vi "בדיקת מפל מתח בין הדקי הממסר תחת עומס Mod.vi"(6 "זרם הדרוש":sgl=20.0, 8 "error":errorcluster, 9 "מפל מתח מקסימלי":dbl=0.205 format="%#_13g", 10 "שם הממסר":string="0410-24534 15A ממסר", 11 "Path for Log":path) -> (0 "error IO":errorcluster, 1 "In Range?":bool, 2 "מפל מתח בין דקי הממסר תחת עומס":dbl, 3 "תוצאה זמנית":dbl)   [LabVIEW 2014]
uses:
  M9700 Driver/86/vi.lib/M9700 Modbus.llb/CTL CMD Register.ctl
  M9700 Driver/85/vi.lib/M9700 Modbus.llb/CTL Register Address.ctl
  <vilib>/Instr/_visa.llb/VISA Configure Serial Port (Instr).vi
  <vilib>/DAQmx/create/channels.llb/DAQmx Create Channel (DO-Digital Output).vi
  <vilib>/DAQmx/write.llb/DAQmx Write (Digital Bool 1Line 1Point).vi
panel:
  out "progress":dbl(slide) min=0.0 max=10.0 scale=0.0..10.0
  in  "stop":bool
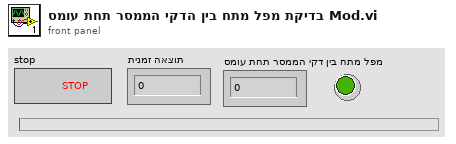
[diagram p1: front panel]
types:
  T1 = enum32{"Invalid", "Standard", "Closed", "Hidden", "Minimized", "Maximized"}
  T2 = typedef "CTL Register Address.ctl" = u16
  T3 = typedef "CTL CMD Register.ctl" = u8
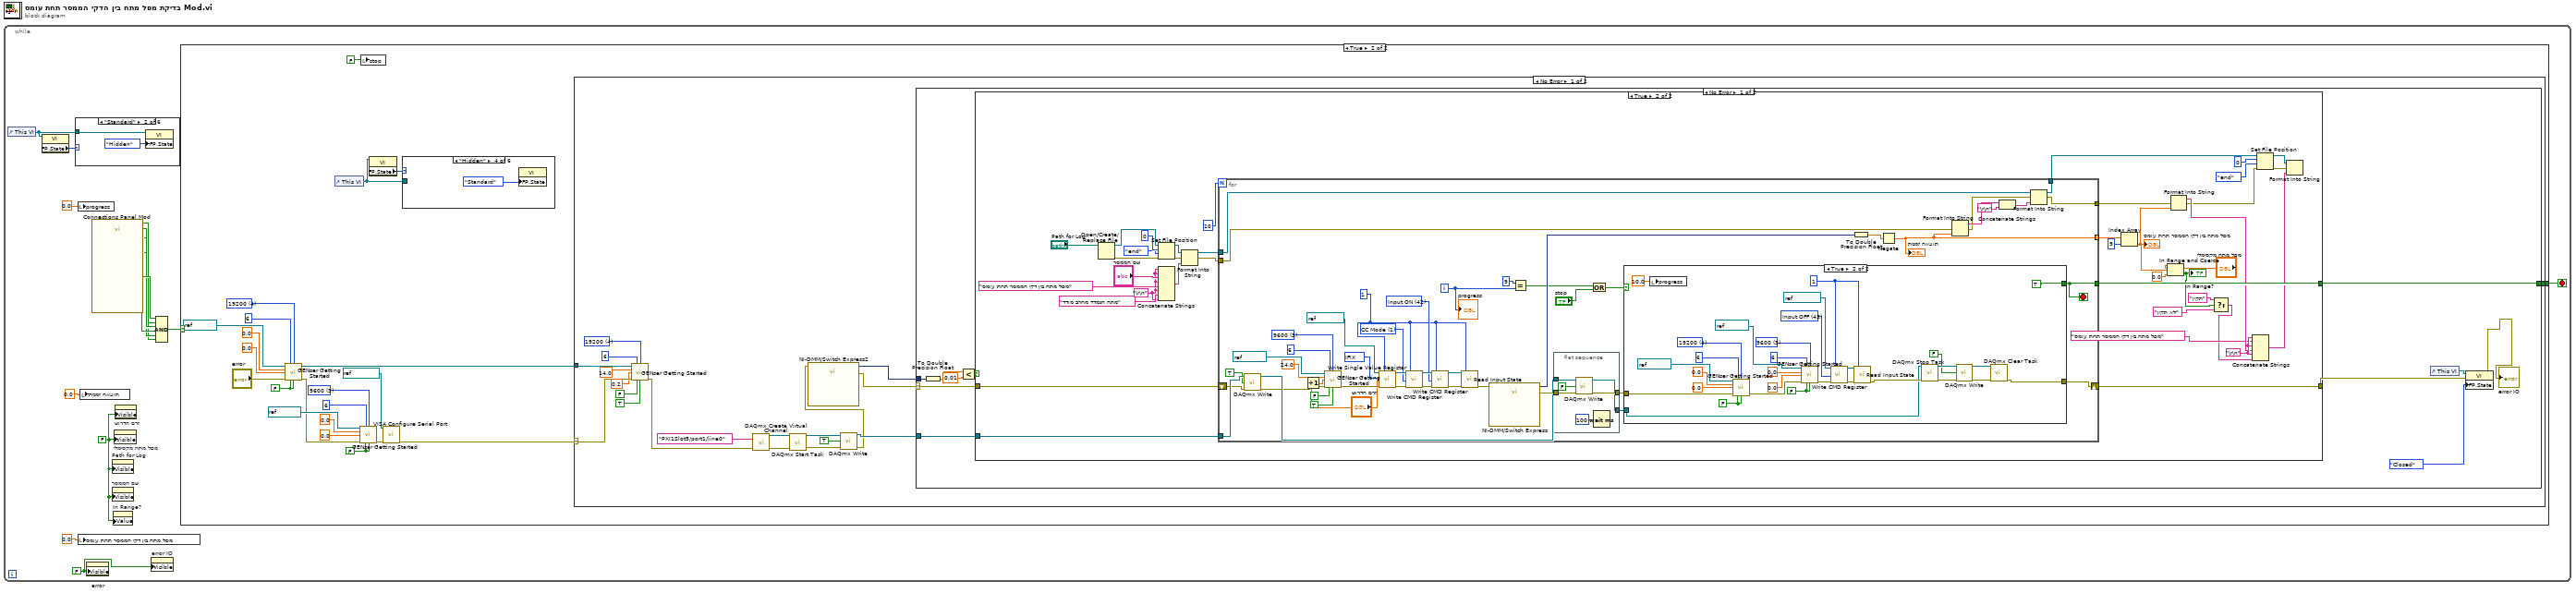
[diagram p0: block diagram]
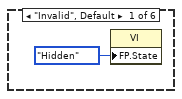
[diagram p2: hidden frame]
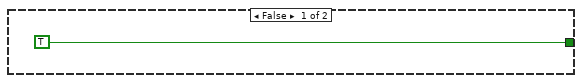
[diagram p7: hidden frame]
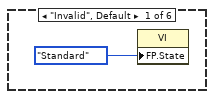
[diagram p8: hidden frame]
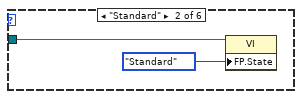
[diagram p9: hidden frame]
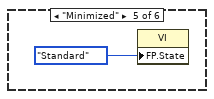
[diagram p11: hidden frame]
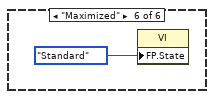
[diagram p12: hidden frame]
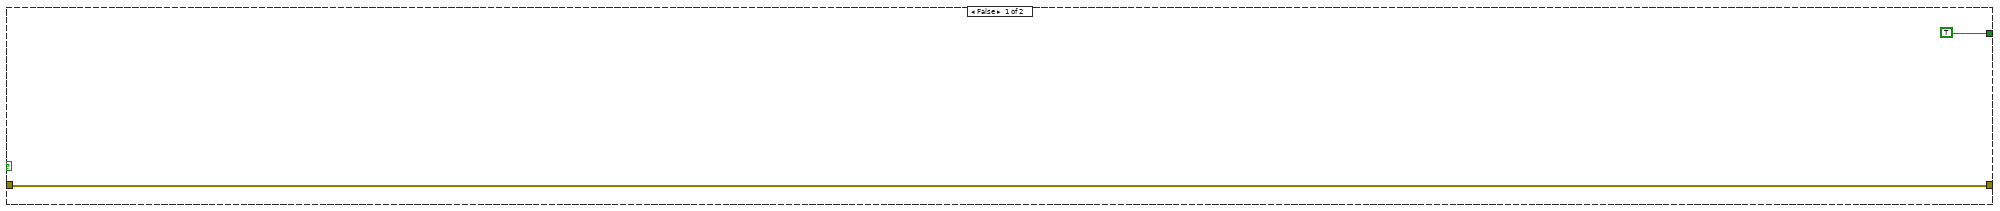
[diagram p13: hidden frame]
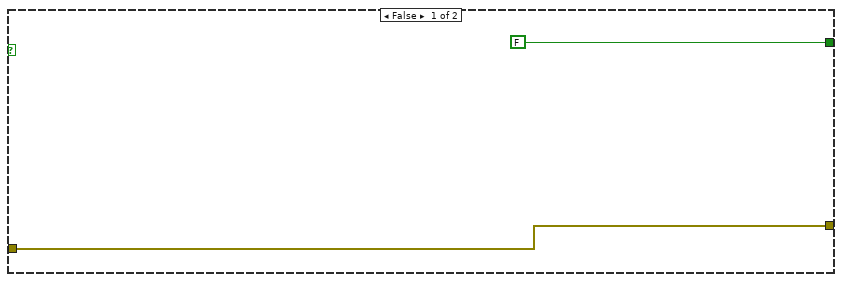
[diagram p14: hidden frame]
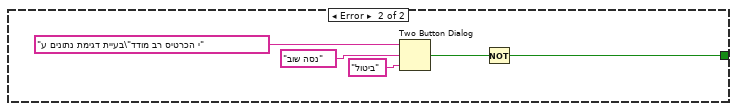
[diagram p15: hidden frame]
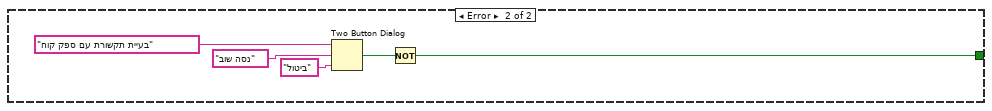
[diagram p16: hidden frame]
diagram:
  n1 = while {
    stop <- w15 stop-if-true
    w1 = FALSE ("Visible")
    w10 = FALSE ("Visible")
    n2 = control-ref of="This VI"() -> (w3:refnum<vi>)
    n3 = property class="VI"(reference=w3) -> ("FP.State"=w2:T1)  [unwired: 1 in, 2 out]
    n4 = case shown="\"Standard\"" w2 {
      tunnel: w3 -> [_ w17 _ _ _ _]
      frame "Invalid", Default {
        n5 = property class="VI"("FP.State"=T1."Hidden" ("Front Panel Window:State")) -> ()  [unwired: 2 in, 2 out]
      }
      frame "Standard" {
        n6 = property class="VI"(reference=w17, "FP.State"=T1."Hidden" ("Front Panel Window:State")) -> ()  [unwired: 1 in, 2 out]
      }
      frame "Closed" {
      }
      frame "Hidden" {
      }
      frame "Minimized" {
      }
      frame "Maximized" {
      }
    }
    n7 = local write "progress"(0.0 ("progress")) -> ()
    n8 = local write "מפל מתח בין דקי הממסר תחת עומס"(0.0 ("מפל מתח בין דקי הממסר תחת עומס")) -> ()
    n9 = local write "תוצאה זמנית"(0.0 ("תוצאה זמנית")) -> ()
    n10 = property on="error" class="Clust (strict)"("Visible"=w10) -> ()  [unwired: 2 in, 2 out]
    n11 = call "Connections Panel Mod.vi"() -> ("Input Name 10"=w4:bool, "Input Name 6"=w8:bool, "Input Name 7"=w7:bool, "Input Name 8"=w6:bool, "Input Name 9"=w5:bool, "OK"=w9:bool)  [unwired: 13 in, 1 out]
    n12 = property on="Path for Log" class="Path"("Visible"=w1) -> ()  [unwired: 2 in, 2 out]
    n13 = property on="שם הממסר" class="Str"("Visible"=w1) -> ()  [unwired: 2 in, 2 out]
    n14 = property on="In Range?" class="Bool (strict)"("Value"=w1) -> ()  [unwired: 2 in, 2 out]
    n15 = property on="מפל מתח מקסימלי" class="DigNum (strict)"("Visible"=w1) -> ()  [unwired: 2 in, 2 out]
    n16 = property on="זרם הדרוש" class="DigNum (strict)"("Visible"=w1) -> ()  [unwired: 2 in, 2 out]
    n17 = property on="error IO" class="Clust (strict)"("Visible"=w10) -> ()  [unwired: 2 in, 2 out]
    n18 = Compound Arithmetic op=AND(w9, w8, w7, w6, w5, w4) -> (w14:bool)
    n19 = case shown="True" w14 {
      tunnel: [TRUE w28] -> w15
      frame False {
      }
      frame True {
        w25 = FALSE ("Reset (T)")
        w33 = u16 3 items=["1200", "2400", "4800", "9600", "19200"] ("BAUD")
        w24 = FALSE ("Output On (T)")
        w38 = u16 4 items=["1200", "2400", "4800", "9600", "19200"] ("BAUD")
        n20 = call "GENser Getting Started.vi"("VISA"=refnum<visa-resource-name> "COM6", "GEN Addr"=i16 6, "BAUD"=w38, "Voltage Limit"=0.0, "Current Limit"=0.0, "error"="error", "Reset (T)"=w24, "Output On (T)"=w24) -> ("VISA out"=w40:refnum<visa-resource-name>, "error out"=w29:errorcluster)  [unwired: 4 in, 2 out]
        n21 = control-ref of="This VI"() -> (w21:refnum<vi>)
        n22 = call "GENser Getting Started.vi"("VISA"=refnum<visa-resource-name> "COM4", "GEN Addr"=i16 6, "BAUD"=w33, "Voltage Limit"=0.0, "Current Limit"=0.0, "error"=w29, "Reset (T)"=w25, "Output On (T)"=w25) -> ("error out"=w26:errorcluster)  [unwired: 4 in, 3 out]
        n23 = local write "stop"(FALSE ("stop")) -> ()
        n24 = property class="VI"(reference=w21) -> ("FP.State"=w22:T1)  [unwired: 1 in, 2 out]
        n25 = call-poly "VISA Configure Serial Port"("VISA resource name"=refnum<visa-resource-name> "COM13", "error in (no error)"=w26) -> ("error out"=w20:errorcluster)  [unwired: 4 in, 9 out]
        n26 = case shown="\"Hidden\"" w22 {
          tunnel: w21 -> [_ w43 _ _ _ _]
          frame "Invalid", Default {
            n27 = property class="VI"("FP.State"=T1."Standard" ("Front Panel Window:State")) -> ()  [unwired: 2 in, 2 out]
          }
          frame "Standard" {
            n28 = property class="VI"(reference=w43, "FP.State"=T1."Standard" ("Front Panel Window:State")) -> ()  [unwired: 1 in, 2 out]
          }
          frame "Closed" {
          }
          frame "Hidden" {
            n29 = property class="VI"("FP.State"=T1."Standard" ("Front Panel Window:State")) -> ()  [unwired: 2 in, 2 out]
          }
          frame "Minimized" {
            n30 = property class="VI"("FP.State"=T1."Standard" ("Front Panel Window:State")) -> ()  [unwired: 2 in, 2 out]
          }
          frame "Maximized" {
            n31 = property class="VI"("FP.State"=T1."Standard" ("Front Panel Window:State")) -> ()  [unwired: 2 in, 2 out]
          }
        }
        n32 = case shown="No Error" w20 {
          selector: w20 -> [w64 _]
          tunnel: w40 -> [w67 _]
          tunnel: [w66 w210] -> w28
          frame No Error {
            w58 = u16 4 items=["1200", "2400", "4800", "9600", "19200"] ("BAUD")
            n33 = call "GENser Getting Started.vi"("VISA"=w67, "GEN Addr"=i16 6, "BAUD"=w58, "Voltage Limit"=14.0, "Current Limit"=0.2, "error"=w64, "Reset (T)"=FALSE, "Output On (T)"=TRUE) -> ("error out"=w49:errorcluster)  [unwired: 4 in, 3 out]
            n34 = call-poly <vilib>:"DAQmx Create Virtual Channel.vi"("lines"=tag "PXI1Slot5/port1/line0", "error in"=w49) -> ("task out"=w56:refnum<k21>, "error out"=w57:errorcluster)  [unwired: 12 in]
            n35 = call <vilib>:"DAQmx Start Task.vi"("task/channels in"=w56, "error in"=w57) -> ("task out"=w54:refnum<k21>, "error out"=w52:errorcluster)  [unwired: 12 in]
            n36 = call-poly <vilib>:"DAQmx Write.vi"("task/channels in"=w54, "data"=TRUE, "error in"=w52) -> ("task out"=w53:refnum<k21>, "error out"=w50:errorcluster)  [unwired: 10 in, 1 out]
            n37 = call "NI-DMM/Switch Express2"("error in"=w50) -> ("signals out"=w65:dynamicdata, "error out"=w48:errorcluster)  [unwired: 16 in, 1 out]
            n38 = case shown="No Error" w48 {
              selector: w48 -> [w76 _]
              tunnel: [w75 w205] -> w66
              tunnel: w65 -> [w78 _]
              tunnel: w53 -> [w69 _]
              frame No Error {
                n39 = To Double Precision Float(number=w78) -> (double precision float=w74:dbl)
                n40 = Less?(x=w74, y=0.01) -> (x < y?=w77:bool)
                n41 = case shown="True" w77 {
                  tunnel: w76 -> [w79 w117]
                  tunnel: [TRUE w118] -> w75
                  tunnel: [w79 w111] -> w70
                  tunnel: w69 -> [_ w112]
                  frame False {
                  }
                  frame True {
                    w96 = "\r\n"
                    w99 = "\r\n"
                    n42 = Open/Create/Replace File(file path (use dialog)="Path for Log") -> (refnum out=w108:refnum<file>, error out=w107:errorcluster)  [unwired: 5 in, 1 out]
                    n43 = Set File Position(offset (in bytes) (0)=i64 0, refnum=w108, from (0:start)=enum16{"start", "end", "current"}."end", error in=w107) -> (refnum out=w103:refnum<file>, error out=w100:errorcluster)
                    n44 = Concatenate Strings(w99, w99, "שם הממסר", w99, "מפל מתח בין דקי הממסר תחת עומס", w99, "מתח הנמדד מהרב מודד", w99) -> (w106:string)
                    n45 = Format Into String(initial string=w103, error in=w100, w106) -> (resulting string=w97:refnum<file>, error out=w98:errorcluster)  [unwired: 1 in]
                    n46 = for {
                      N: 10 -> [_]
                      tunnel: [w150] -> w118
                      shift-right: [w147] -> w111
                      shift-left: w117 -> [w142]
                      tunnel: [w122] -> w116 mode=indexing
                      tunnel: w112 -> [w143]
                      tunnel: w98 -> [w132]
                      tunnel: w97 -> [w134]
                      tunnel: [w131] -> w90
                      tunnel: [w130] -> w81
                      i -> [w146]
                      stop <- w150 stop-if-true
                      w126 = T2 2561 items=["REMOTE"=1283, "ISTATE"=1296, "CMD"=2560, "IFIX"=2561, "UFIX"=2563, "PFIX"=2565, "RFIX"=2567, "IMAX"=2612, "UMAX"=2614, "PMAX"=2616, "U"=2816, "I"=2818, "MODEL"=2822, "EDITION"=2823] ("Register Address")
                      w127 = T3 42 items=["CC Mode"=1, "CV Mode"=2, "CW Mode"=3, "CR Mode"=4, "Short Mode"=26, "Set SysPara"=41, "Input ON"=42, "Input OFF"=43] ("CMD Register Value")
                      w120 = u8 1 ("Load Address")
                      w121 = T3 1 items=["CC Mode"=1, "CV Mode"=2, "CW Mode"=3, "CR Mode"=4, "Short Mode"=26, "Set SysPara"=41, "Input ON"=42, "Input OFF"=43] ("CMD Register Value")
                      w165 = u16 3 items=["1200", "2400", "4800", "9600", "19200"] ("BAUD")
                      n47 = call-poly <vilib>:"DAQmx Write.vi"("task/channels in"=w143, "data"=TRUE, "error in"=w142) -> ("task out"=w141:refnum<k21>, "error out"=w140:errorcluster)  [unwired: 10 in, 1 out]
                      n48 = Increment(x="זרם הדרוש") -> (x+1=w125:sgl)
                      n49 = call "GENser Getting Started.vi"("VISA"=refnum<visa-resource-name> "COM4", "GEN Addr"=i16 6, "BAUD"=w165, "Voltage Limit"=24.0, "Current Limit"=w125, "error"=w140, "Reset (T)"=FALSE, "Output On (T)"=TRUE) -> ("error out"=w159:errorcluster)  [unwired: 4 in, 3 out]
                      n50 = call "Write Single Value Register.vi"("VISA resource name"=refnum<visa-resource-name> "COM13", "Starting Address(HEX)"=w126, "Register Single Value"="זרם הדרוש", "error in"=w159, "Load Address"=w120) -> ("VISA resource name out"=w161:refnum<visa-resource-name>, "error out"=w160:errorcluster)  [unwired: 13 out]
                      n51 = call "Write CMD Register.vi"("VISA resource name"=w161, "CMD Value"=w121, "error in"=w160, "Load Address"=w120) -> ("VISA resource name out"=w128:refnum<visa-resource-name>, "error out"=w158:errorcluster)  [unwired: 14 in]
                      n52 = call "Write CMD Register.vi"("VISA resource name"=w128, "CMD Value"=w127, "error in"=w158, "Load Address"=w120) -> ("VISA resource name out"=w129:refnum<visa-resource-name>, "error out"=w157:errorcluster)  [unwired: 14 in]
                      n53 = call "Read Input State.vi"("VISA resource name"=w129, "error in"=w157, "Load Address"=w120) -> ("error out"=w156:errorcluster)  [unwired: 16 out]
                      n54 = call "NI-DMM/Switch Express"("error in"=w156) -> ("signals out"=w155:dynamicdata, "error out"=w144:errorcluster)  [unwired: 16 in, 1 out]
                      n55 = Equal?(x=9, y=w146) -> (x = y?=w152:bool)
                      n56 = flat-sequence {
                        tunnel: [w172] -> w145
                        tunnel: w144 -> [w171]
                        tunnel: w141 -> [w169]
                        tunnel: [w168] -> w138
                        frame #0 {
                          n57 = call-poly <vilib>:"DAQmx Write.vi"("task/channels in"=w169, "data"=FALSE, "error in"=w171) -> ("task out"=w168:refnum<k21>, "error out"=w172:errorcluster)  [unwired: 10 in, 1 out]
                          n58 = Wait (ms)(milliseconds to wait=u32 100) -> ()  [unwired: 1 out]
                        }
                      }
                      n59 = Or(x=w152, y="stop") -> (x .or. y?=w153:bool)
                      n60 = case shown="True" w153 {
                        tunnel: [FALSE TRUE] -> w150
                        tunnel: w145 -> [w173 w193]
                        tunnel: [w173 w177] -> w147
                        tunnel: w138 -> [_ w179]
                        frame False {
                        }
                        frame True {
                          w175 = u8 1 ("Load Address")
                          w176 = T3 43 items=["CC Mode"=1, "CV Mode"=2, "CW Mode"=3, "CR Mode"=4, "Short Mode"=26, "Set SysPara"=41, "Input ON"=42, "Input OFF"=43] ("CMD Register Value")
                          w191 = FALSE ("Reset (T)")
                          w197 = u16 3 items=["1200", "2400", "4800", "9600", "19200"] ("BAUD")
                          w190 = FALSE ("Reset (T)")
                          w200 = u16 4 items=["1200", "2400", "4800", "9600", "19200"] ("BAUD")
                          n61 = local write "progress"(10.0 ("progress")) -> ()
                          n62 = call "GENser Getting Started.vi"("VISA"=refnum<visa-resource-name> "COM6", "GEN Addr"=i16 6, "BAUD"=w200, "Voltage Limit"=0.0, "Current Limit"=0.0, "error"=w193, "Reset (T)"=w190, "Output On (T)"=w190) -> ("error out"=w192:errorcluster)  [unwired: 4 in, 3 out]
                          n63 = call "GENser Getting Started.vi"("VISA"=refnum<visa-resource-name> "COM4", "GEN Addr"=i16 6, "BAUD"=w197, "Voltage Limit"=0.0, "Current Limit"=0.0, "error"=w192, "Reset (T)"=w191, "Output On (T)"=w191) -> ("error out"=w189:errorcluster)  [unwired: 4 in, 3 out]
                          n64 = call "Write CMD Register.vi"("VISA resource name"=refnum<visa-resource-name> "COM13", "CMD Value"=w176, "error in"=w189, "Load Address"=w175) -> ("VISA resource name out"=w178:refnum<visa-resource-name>, "error out"=w188:errorcluster)  [unwired: 14 in]
                          n65 = call "Read Input State.vi"("VISA resource name"=w178, "error in"=w188, "Load Address"=w175) -> ("error out"=w180:errorcluster)  [unwired: 16 out]
                          n66 = call <vilib>:"DAQmx Stop Task.vi"("task/channels in"=w179, "error in"=w180) -> ("task out"=w185:refnum<k21>, "error out"=w183:errorcluster)  [unwired: 12 in]
                          n67 = call-poly <vilib>:"DAQmx Write.vi"("task/channels in"=w185, "data"=FALSE, "error in"=w183) -> ("task out"=w182:refnum<k21>, "error out"=w181:errorcluster)  [unwired: 10 in, 1 out]
                          n68 = call <vilib>:"DAQmx Clear Task.vi"("task in"=w182, "error in"=w181) -> ("error out"=w177:errorcluster)  [unwired: 13 in]
                        }
                      }
                      n69 = To Double Precision Float(number=w155) -> (double precision float=w123:dbl)
                      n70 = Negate(x=w123) -> (-x=w122:dbl)
                      "תוצאה זמנית" <- w122
                      n71 = Format Into String(error in=w132, w122) -> (resulting string=w136:string, error out=w133:errorcluster)  [unwired: 2 in]
                      n72 = Concatenate Strings(w136, "\r\n") -> (w135:string)
                      n73 = Format Into String(initial string=w134, error in=w133, w135) -> (resulting string=w131:refnum<file>, error out=w130:errorcluster)  [unwired: 1 in]
                      "progress" <- w146
                    }
                    n74 = Index Array(array=w116, index=9) -> (element=w89:dbl)
                    "מפל מתח בין דקי הממסר תחת עומס" <- w89
                    n75 = In Range and Coerce(upper limit="מפל מתח מקסימלי", x=w89, lower limit=0.0) -> (In Range?=w84:bool)  [unwired: 1 out]
                    "In Range?" <- w84
                    n76 = Format Into String(error in=w81, w89) -> (resulting string=w88:string, error out=w82:errorcluster)  [unwired: 2 in]
                    n77 = Select(t="תקין", s=w84, f="לא תקין") -> (s? t:f=w83:string)
                    n78 = Concatenate Strings(w96, "מפל מתח בין דקי הממסר תחת עומס" ("string"), w96, w88, w96, w83) -> (w91:string)
                    n79 = Set File Position(offset (in bytes) (0)=i64 0, refnum=w90, from (0:start)=enum16{"start", "end", "current"}."end", error in=w82) -> (refnum out=w93:refnum<file>, error out=w92:errorcluster)
                    n80 = Format Into String(initial string=w93, error in=w92, w91) -> ()  [unwired: 1 in, 2 out]
                  }
                }
                n81 = control-ref of="This VI"() -> (w72:refnum<vi>)
                n82 = property class="VI"(reference=w72, error in=w70, "FP.State"=T1."Closed" ("Front Panel Window:State")) -> (error out=→"error IO":errorcluster)  [unwired: 1 out]
              }
              frame Error {
                n83 = Two Button Dialog(message="בעיית דגימת נתונים ע\"י הכרטיס רב מודד", 1:"ביטול" ("F button name (\"Cancel\")"), 2:"נסה שוב" ("T button name (\"OK\")")) -> (T button?=w206:bool)
                n84 = Not(x=w206) -> (.not. x?=w205:bool)
              }
            }
          }
          frame Error {
            n85 = Two Button Dialog(message="בעיית תקשורת עם ספק קוח", 1:"ביטול" ("F button name (\"Cancel\")"), 2:"נסה שוב" ("T button name (\"OK\")")) -> (T button?=w211:bool)
            n86 = Not(x=w211) -> (.not. x?=w210:bool)
          }
        }
      }
    }
  }
